vi "onStarted.vi"(8 "error in (no error)":errorcluster, 11 "DAQ":refnum<class "DAQ.lvclass">) -> (0 "error out":errorcluster, 3 "DAQ out":refnum<class "DAQ.lvclass">)   [LabVIEW 2016, in "DAQ.lvclass"]
doc: "JKI State Machine Objects (SMO) 1.2.1.55\nJKI - JKI\nCopyright (c) 2017, JKI"
uses:
  DAQ.lvclass
  DAQ.lvclass/DAQ.ctl
  <vilib>/JKI/JKI SMO/SMO/SMO.lvclass
panel:
  # "For instructions on how to use the JKI State Machine Objects, examples and video tutorials, visit:\nhttp://jki.net/state-machine-objects/\n\nJKI State Machine Objects™\nhttp://jki.net/state-machine-objects/\nCopyright (C) 2005-2015, JKI <info@jki.net>\nALL RIGHTS RESERVED"
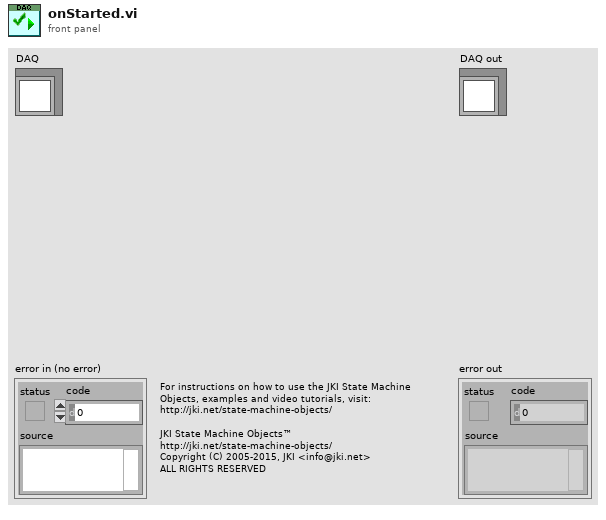
[diagram p1: front panel]
types:
  T1 = typedef "DAQ.lvclass/PrivateEvents--DAQ.AI.Channels.ctl" = string
  T2 = typedef "DAQ.lvclass/PrivateEvents--DAQ.AO.Channels.ctl" = string
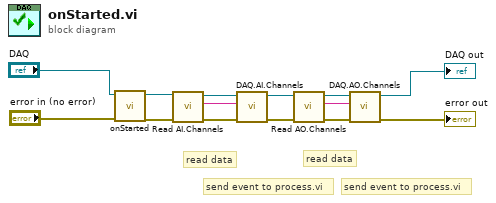
[diagram p0: block diagram]
diagram:
  # "send event to process.vi"
  # "read data"
  # "send event to process.vi"
  # "read data"
  n1 = call-parent "onStarted.vi"("error in (no error)"="error in (no error)", "SMO"="DAQ") -> ("error out"=w2:errorcluster, "SMO out"=w10:refnum<class "DAQ.lvclass">)  [unwired: 8 in]
  n2 = call "Read AI.Channels.vi"("error in (no error)"=w2, "DAQ in"=w10) -> ("error out"=w3:errorcluster, "AI.Channels"=w1:T1, "DAQ out"=w9:refnum<class "DAQ.lvclass">)  [unwired: 7 in]
  n3 = call "DAQ.AI.Channels.vi"("error in (no error)"=w3, "AI.Channels"=w1, "DAQ"=w9) -> ("error out"=w4:errorcluster, "DAQ out"=w8:refnum<class "DAQ.lvclass">)  [unwired: 7 in]
  n4 = call "Read AO.Channels.vi"("error in (no error)"=w4, "DAQ in"=w8) -> ("error out"=w5:errorcluster, "AO.Channels"=w6:T2, "DAQ out"=w7:refnum<class "DAQ.lvclass">)  [unwired: 7 in]
  n5 = call "DAQ.AO.Channels.vi"("error in (no error)"=w5, "AO.Channels"=w6, "DAQ"=w7) -> ("error out"=→"error out":errorcluster, "DAQ out"=→"DAQ out":refnum<class "DAQ.lvclass">)  [unwired: 7 in]
